vi "Define Test Suite (JUnit Report).vi"(6 "Verbose (F)":bool, 8 "error in (no error)":errorcluster, 9 "Report Path":path, 10 "Interactive":bool, 11 "Label (VI Title)":string) -> (0 "error out":errorcluster, 3 "Test Suite":refnum<class "Test Suite.lvclass">)   [LabVIEW 2013, in "Caraya.lvlib" / "Test Suite.lvclass"]
doc: "Registers the calling VI as a test suite. If Interactive is True, the interactive user interface is opened when the test suite is executed. If the Report Path is set, a report file will be generated with the test results.\n\n--\nCopyright © 2015 JKI All rights reserved.\n\nAuthor: Tomi Maila <tomi.maila@jki.net>\n\nThis library is provided \"AS IS\" ,WITHOUT WARRANTIES OR\nCONDITIONS OF ANY KIND, either express or implied.\n\nJKI -- jki.net"
uses:
  Test Suite.lvclass
  Test Assert Factory/Test Assert Factory.lvclass
  Test Report.JUnit/Test Report.JUnit.lvclass
  subVIs/Test Notification.ctl
  Test Report/Test Report.lvclass/Test Report.ctl
  Test Assert Factory/Test Assert Factory.lvclass/Test Assert Factory.ctl
  Assert Factory/Assert Factory.lvclass
  Test Suite.lvclass/Test Suite.ctl
  Test Manager/Test Manager.lvclass
  Caraya.lvlib
  Assert Factory Manager/Assert Factory Manager.lvclass
  Test Report/Test Report.lvclass
panel:
  # "Copyright © 2015 JKI All rights reserved.\n\nAuthor: Tomi Maila <tomi.maila@jki.net>\n\nThis library is provided \"AS IS\" ,WITHOUT WARRANTIES OR\nCONDITIONS OF ANY KIND, either express or implied.\n\nJKI -- jki.net"
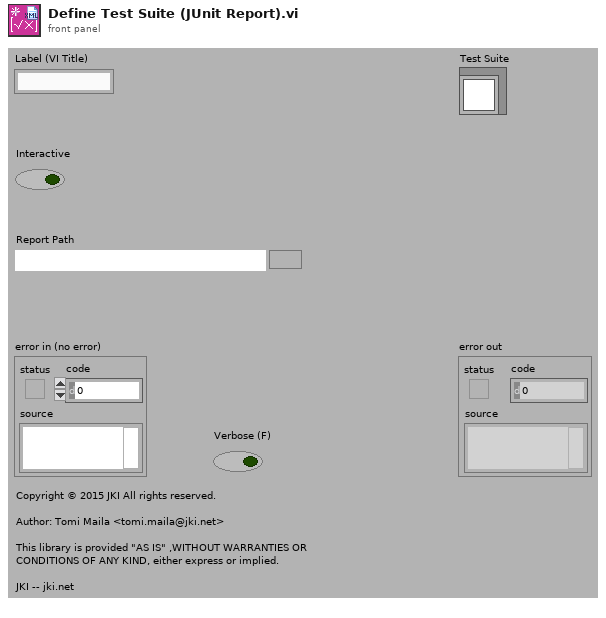
[diagram p1: front panel]
types:
  T1 = typedef "Caraya.lvlib/Test Notification.ctl" = bool
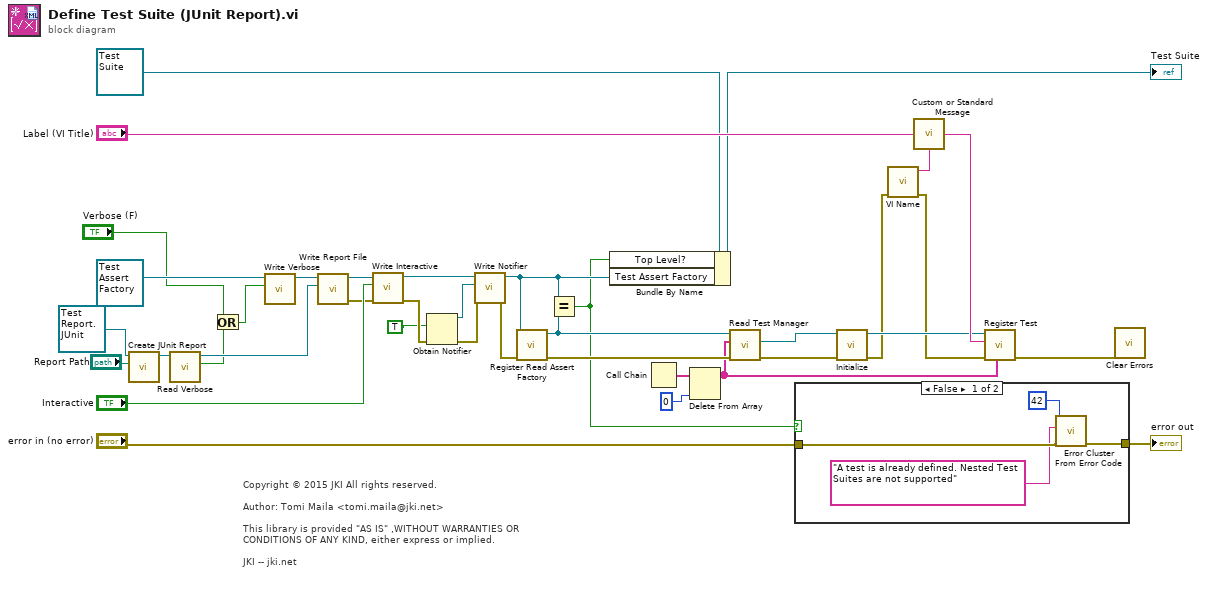
[diagram p0: block diagram]
diagram:
  # "Copyright © 2015 JKI All rights reserved.\n\nAuthor: Tomi Maila <tomi.maila@jki.net>\n\nThis library is provided \"AS IS\" ,WITHOUT WARRANTIES OR\nCONDITIONS OF ANY KIND, either express or implied.\n\nJKI -- jki.net"
  n1 = call "Create JUnit Report.vi"("Report Path"="Report Path", "Test Report.JUnit in"=refnum<class "Test Report.JUnit.lvclass"> refnum) -> ("Test Report.JUnit out"=w6:refnum<class "Test Report.JUnit.lvclass">)  [unwired: 8 in, 1 out]
  n2 = call "Read Verbose.vi"("Test Report in"=w6) -> ("Verbose"=w4:bool, "Test Report out"=w5:refnum<class "Test Report.JUnit.lvclass">)  [unwired: 8 in, 1 out]
  n3 = Or(x="Verbose (F)", y=w4) -> (x .or. y?=w2:bool)
  n4 = call "Write Verbose.vi"("Verbose"=w2, "Test Assert Factory in"=refnum<class "Test Assert Factory.lvclass"> refnum ("Caraya.lvlib:Test Assert Factory.lvclass")) -> ("Test Assert Factory out"=w7:refnum<class "Test Assert Factory.lvclass">)  [unwired: 8 in, 1 out]
  n5 = call "Write Report File.vi"("Test Report"=w5, "Test Assert Factory in"=w7) -> ("error out"=w34:errorcluster, "Test Assert Factory out"=w36:refnum<class "Test Assert Factory.lvclass">)  [unwired: 8 in]
  n6 = call "Write Interactive.vi"("error in (no error)"=w34, "Interactive"="Interactive", "Test Assert Factory in"=w36) -> ("error out"=w29:errorcluster, "Test Assert Factory out"=w32:refnum<class "Test Assert Factory.lvclass">)  [unwired: 7 in]
  n7 = Obtain Notifier(notification data type=T1 TRUE ("Test"), error in (no error)=w29) -> (notifier out=w27:refnum<notifier>, error out=w28:errorcluster)  [unwired: 2 in, 1 out]
  n8 = call "Write Notifier.vi"("error in (no error)"=w28, "notifier"=w27, "Test Assert Factory in"=w32) -> ("error out"=w33:errorcluster, "Test Assert Factory out"=w16:refnum<class "Test Assert Factory.lvclass">)  [unwired: 7 in]
  n9 = call "Register Read Assert Factory.vi"("error in (no error)"=w33, "Assert Factory"=w16) -> ("error out"=w37:errorcluster, "Assert Factory"=w15:refnum<class "Assert Factory.lvclass">)  [unwired: 8 in]
  n10 = Equal?(x=w16, y=w15) -> (x = y?=w12:bool)
  n11 = Bundle By Name(cluster=refnum<class "Test Suite.lvclass"> refnum ("Test Suite"), "Top Level?"=w12, "Test Assert Factory"=w16) -> (→"Test Suite":refnum<class "Test Suite.lvclass">)
  n12 = Call Chain() -> (call chain=w18:string[])
  n13 = Delete From Array(array=w18, index=0) -> (array with subset deleted=w17:string[])  [unwired: 1 in, 1 out]
  n14 = call-dynamic "Read Test Manager.vi"("error in (no error)"=w37, "VI Call Chain"=w17, "Assert Factory in"=w15) -> ("error out"=w23:errorcluster, "Test Manager"=w11:refnum<class "Test Manager.lvclass">)  [unwired: 6 in, 1 out]
  n15 = case shown="False" w12 {
    tunnel: [w42 w43] -> w14
    tunnel: "error in (no error)" -> [w41 w43]
    frame False {
      n16 = call <vilib>:"Error Cluster From Error Code.vi"("error in (no error)"=w41, "error message (\"\")"="A test is already defined. Nested Test Suites are not supported" ("error message (\"\")"), "error code (0)"=42) -> ("error out"=w42:errorcluster)  [unwired: 6 in]
    }
    frame True {
    }
  }
  "error out" <- w14
  n17 = call-dynamic "Initialize.vi"("error in (no error)"=w23, "Test Manager in"=w11) -> ("error out"=w22:errorcluster, "Test Manager out"=w24:refnum<class "Test Manager.lvclass">)  [unwired: 8 in]
  n18 = call "VI Name.vi"("error in (no error)"=w22) -> ("error out"=w21:errorcluster, "VI Name"=w26:string)  [unwired: 9 in]
  n19 = call "Custom or Standard Message.vi"("Custom Message"="Label (VI Title)", "Standard Message"=w26) -> ("Message"=w25:string)
  n20 = call-dynamic "Register Test.vi"("Call Chain"=w17, "error in (no error)"=w21, "Name"=w25, "Test Manager in"=w24) -> ("error out"=w20:errorcluster)  [unwired: 6 in, 1 out]
  n21 = call <vilib>:"Clear Errors.vi"("error in (no error)"=w20) -> ()  [unwired: 6 in, 1 out]
